vi "Mirror_GUI.vi"(10 "stop 2":refnum<vi>, 11 "GUI_cluster":T1={"Sub Panel"=refnum, "GUIdevice"="Bella_LP_Mode", "CtlRef"=refnum, "User Event in"=refnum}) -> ()   [LabVIEW 2020]
uses:
  Shared/GUI_Template/GUI_master/tcp new data cluster.ctl
  General GUIs/General-Controler/firstCall_TypDef.ctl
  Controls/eventtypdef1.ctl
  Controls/GUI_cluster.ctl
panel:
  out "UDP error message":string
  out "status ref":refnum<vi>[](array[refnum])
  out "pathRef":refnum<vi>[](array[refnum])
  in  "pushSave":bool
  out "Page Label":string="StagingTRA1"
  in  "save::4":bool caption="save"
  in  "save::3":bool caption="save"
  in  "save::2":bool caption="save"
  in  "save::1":bool caption="save"
  in  "LocalSavingPath::4":path=path "Z:/5_resources/StagingResources/TRAposition/testNEW" caption="LocalSavingPath::1"
  in  "LocalSavingPath::3":path=path "Z:/5_resources/StagingResources/TRAposition/testNEW" caption="LocalSavingPath::1"
  in  "LocalSavingPath::2":path=path "Z:/5_resources/StagingResources/TRAposition/testNEW" caption="LocalSavingPath::1"
  in  "LocalSavingPath::1":path=path "Z:/5_resources/StagingResources/TRAposition/testNEW"
  in  "save":bool
  out "GUIdevice 3":string="StagingTRA3"
  out "GUIdevice 4":string="TREX TRA1"
  out "error out":errorcluster
  out "GUIdevice 2":string="StagingTRA2"
  in  "Tab Control":T2(tab)
  in  "StepSize::1":dbl=0.01 caption="StepSize" min=-1.0 max=1.0 format="%#_2p"
  in  "Cluster 20":T3
  in  "Y":T4={"position::1"=2.74161, "Channel::1"=enum."Axis 2", "Status::1"=enum."DISABLE"} {"position::1" min=0.0 max=6.0 format="%#_8g"}
  in  "X":T5={"position::1"=3.02685, "Channel::1"=enum."Axis 1", "Status::1"=enum."DISABLE"} {"position::1" min=0.0 max=6.0 format="%#_8g"}
  in  "Cluster 40":T6
  in  "Cluster 50":T7
  in  "Cluster 30":T8
  out "device status::1":string="Initialized" caption="Device status"
  in  "<command>::1":bool
  in  "StepSize::2":dbl=0.01 caption="StepSize" min=-1.0 max=1.0 format="%#_2p"
  in  "Cluster 23":T9
  in  "Y":T10={"position::2"=3.24237, "Channel::2"=enum."Axis 2", "Status::2"=enum."DISABLE"} {"position::2" min=0.0 max=6.0 format="%#_8g"}
  in  "X":T11={"position::2"=2.27011, "Channel::2"=enum."Axis 1", "Status::2"=enum."DISABLE"} {"position::2" min=0.0 max=6.0 format="%#_8g"}
  in  "Cluster 43":T12
  in  "Cluster 53":T13
  in  "Cluster 33":T14
  out "device status::2":string="Initialized" caption="Device status"
  in  "<command>::2":bool
  in  "StepSize::3":dbl=0.01 caption="StepSize" min=-1.0 max=1.0 format="%#_2p"
  in  "Cluster 22":T15
  in  "Y":T16={"position::3"=5.00224, "Channel::3"=enum."Axis 2", "Status::3"=enum."DISABLE"} {"position::3" min=0.0 max=0.0 format="%#_8g"}
  in  "X":T17={"position::3"=1.52721, "Channel::3"=enum."Axis 1", "Status::3"=enum."DISABLE"} {"position::3" min=0.0 max=0.0 format="%#_8g"}
  in  "Cluster 42":T18
  in  "Cluster 52":T19
  in  "Cluster 32":T20
  out "device status::3":string="Initialized" caption="Device status"
  in  "<command>::3":bool
  in  "StepSize::4":dbl=0.01 caption="StepSize" min=-1.0 max=1.0 format="%#_2p"
  in  "Cluster 21":T21
  in  "Y":T22={"position::4"=4.68088, "Channel::4"=enum."Axis 2", "Status::4"=enum."DISABLE"} {"position::4" min=0.0 max=6.0 format="%#_8g"}
  in  "X":T23={"position::4"=0.99394, "Channel::4"=enum."Axis 1", "Status::4"=enum."DISABLE"} {"position::4" min=0.0 max=6.0 format="%#_8g"}
  in  "Cluster 41":T24
  in  "Cluster 51":T25
  in  "Cluster 31":T26
  out "device status::4":string="Initialized" caption="Device status"
  in  "<command>::4":bool
  in  "Mirror":T27(ring)
  out "GUIdevice 1":string="StagingTRA1"
  in  "stop":bool
  in  "Refresh Button":bool
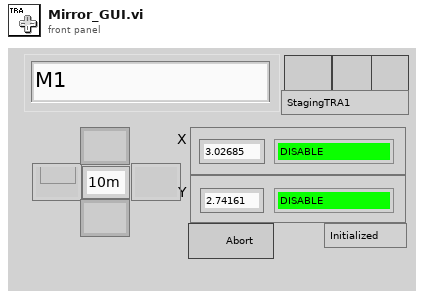
[diagram p1: front panel]
types:
  T1 = typedef "GUI_cluster.ctl" = cluster{"Sub Panel":refnum<vi>, "GUIdevice":string, "CtlRef":refnum<vi>, "User Event in":refnum<user-event>}
  T2 = enum32{"StagingTRA1", "StagingTRA2", "StagingTRA3", "TREX TRA1"}
  T3 = cluster{"relativeMovePos::1":bool, "Channel::1":enum16{"Axis 1", "Axis 3", "Axis 5"}}
  T4 = cluster{"position::1":dbl, "Channel::1":enum16{"Axis 2", "Axis 4", "Axis 6"}, "Status::1":enum16{"NOT REFERENCED", "CONFIGURATION", "HOMING", "MOVING", "READY", "DISABLE", "JOGGING"}}
  T5 = cluster{"position::1":dbl, "Channel::1":enum16{"Axis 1", "Axis 3", "Axis 5"}, "Status::1":enum16{"NOT REFERENCED", "CONFIGURATION", "HOMING", "MOVING", "READY", "DISABLE", "JOGGING"}}
  T6 = cluster{"relativeMovePos::1":bool, "Channel::1":enum16{"Axis 2", "Axis 4", "Axis 6"}}
  T7 = cluster{"relativeMoveNeg::1":bool, "Channel::1":enum16{"Axis 2", "Axis 4", "Axis 6"}}
  T8 = cluster{"relativeMoveNeg::1":bool, "Channel::1":enum16{"Axis 1", "Axis 3", "Axis 5"}}
  T9 = cluster{"relativeMovePos::2":bool, "Channel::2":enum16{"Axis 1", "Axis 3", "Axis 5"}}
  T10 = cluster{"position::2":dbl, "Channel::2":enum16{"Axis 2", "Axis 4", "Axis 6"}, "Status::2":enum16{"NOT REFERENCED", "CONFIGURATION", "HOMING", "MOVING", "READY", "DISABLE", "JOGGING"}}
  T11 = cluster{"position::2":dbl, "Channel::2":enum16{"Axis 1", "Axis 3", "Axis 5"}, "Status::2":enum16{"NOT REFERENCED", "CONFIGURATION", "HOMING", "MOVING", "READY", "DISABLE", "JOGGING"}}
  T12 = cluster{"relativeMovePos::2":bool, "Channel::2":enum16{"Axis 2", "Axis 4", "Axis 6"}}
  T13 = cluster{"relativeMoveNeg::2":bool, "Channel::2":enum16{"Axis 2", "Axis 4", "Axis 6"}}
  T14 = cluster{"relativeMoveNeg::2":bool, "Channel::2":enum16{"Axis 1", "Axis 3", "Axis 5"}}
  T15 = cluster{"relativeMovePos::3":bool, "Channel::3":enum16{"Axis 1", "Axis 3", "Axis 5"}}
  T16 = cluster{"position::3":dbl, "Channel::3":enum16{"Axis 2", "Axis 4", "Axis 6"}, "Status::3":enum16{"NOT REFERENCED", "CONFIGURATION", "HOMING", "MOVING", "READY", "DISABLE", "JOGGING"}}
  T17 = cluster{"position::3":dbl, "Channel::3":enum16{"Axis 1", "Axis 3", "Axis 5"}, "Status::3":enum16{"NOT REFERENCED", "CONFIGURATION", "HOMING", "MOVING", "READY", "DISABLE", "JOGGING"}}
  T18 = cluster{"relativeMovePos::3":bool, "Channel::3":enum16{"Axis 2", "Axis 4", "Axis 6"}}
  T19 = cluster{"relativeMoveNeg::3":bool, "Channel::3":enum16{"Axis 2", "Axis 4", "Axis 6"}}
  T20 = cluster{"relativeMoveNeg::3":bool, "Channel::3":enum16{"Axis 1", "Axis 3", "Axis 5"}}
  T21 = cluster{"relativeMovePos::4":bool, "Channel::4":enum16{"Axis 1", "Axis 3", "Axis 5"}}
  T22 = cluster{"position::4":dbl, "Channel::4":enum16{"Axis 2", "Axis 4", "Axis 6"}, "Status::4":enum16{"NOT REFERENCED", "CONFIGURATION", "HOMING", "MOVING", "READY", "DISABLE", "JOGGING"}}
  T23 = cluster{"position::4":dbl, "Channel::4":enum16{"Axis 1", "Axis 3", "Axis 5"}, "Status::4":enum16{"NOT REFERENCED", "CONFIGURATION", "HOMING", "MOVING", "READY", "DISABLE", "JOGGING"}}
  T24 = cluster{"relativeMovePos::4":bool, "Channel::4":enum16{"Axis 2", "Axis 4", "Axis 6"}}
  T25 = cluster{"relativeMoveNeg::4":bool, "Channel::4":enum16{"Axis 2", "Axis 4", "Axis 6"}}
  T26 = cluster{"relativeMoveNeg::4":bool, "Channel::4":enum16{"Axis 1", "Axis 3", "Axis 5"}}
  T27 = enum16{"M1", "BS", "M3", "OAP1", "M4", "OAP2", "M5", "n/a", "n/a ", "M20", "SIM", "M22"}
  T28 = typedef "eventtypdef1.ctl" = cluster{"label":string, "Sub Panel":refnum<vi>, "CtlRef":refnum<vi>, "This VI":refnum<vi>}
  T29 = typedef "tcp new data cluster.ctl" = cluster{"EventEnum":enum16{"new data", "connection status update"}, "Device name":string}
  T30 = typedef "firstCall_TypDef.ctl" = enum16{"reset", "read"}
  T31 = typedef "LVFontTypeDef.ctl" = cluster{"Font Name":string, "Size":u16, "Bold":bool, "Italic":bool, "Underline":bool, "Strikeout":bool, "Color":u32}
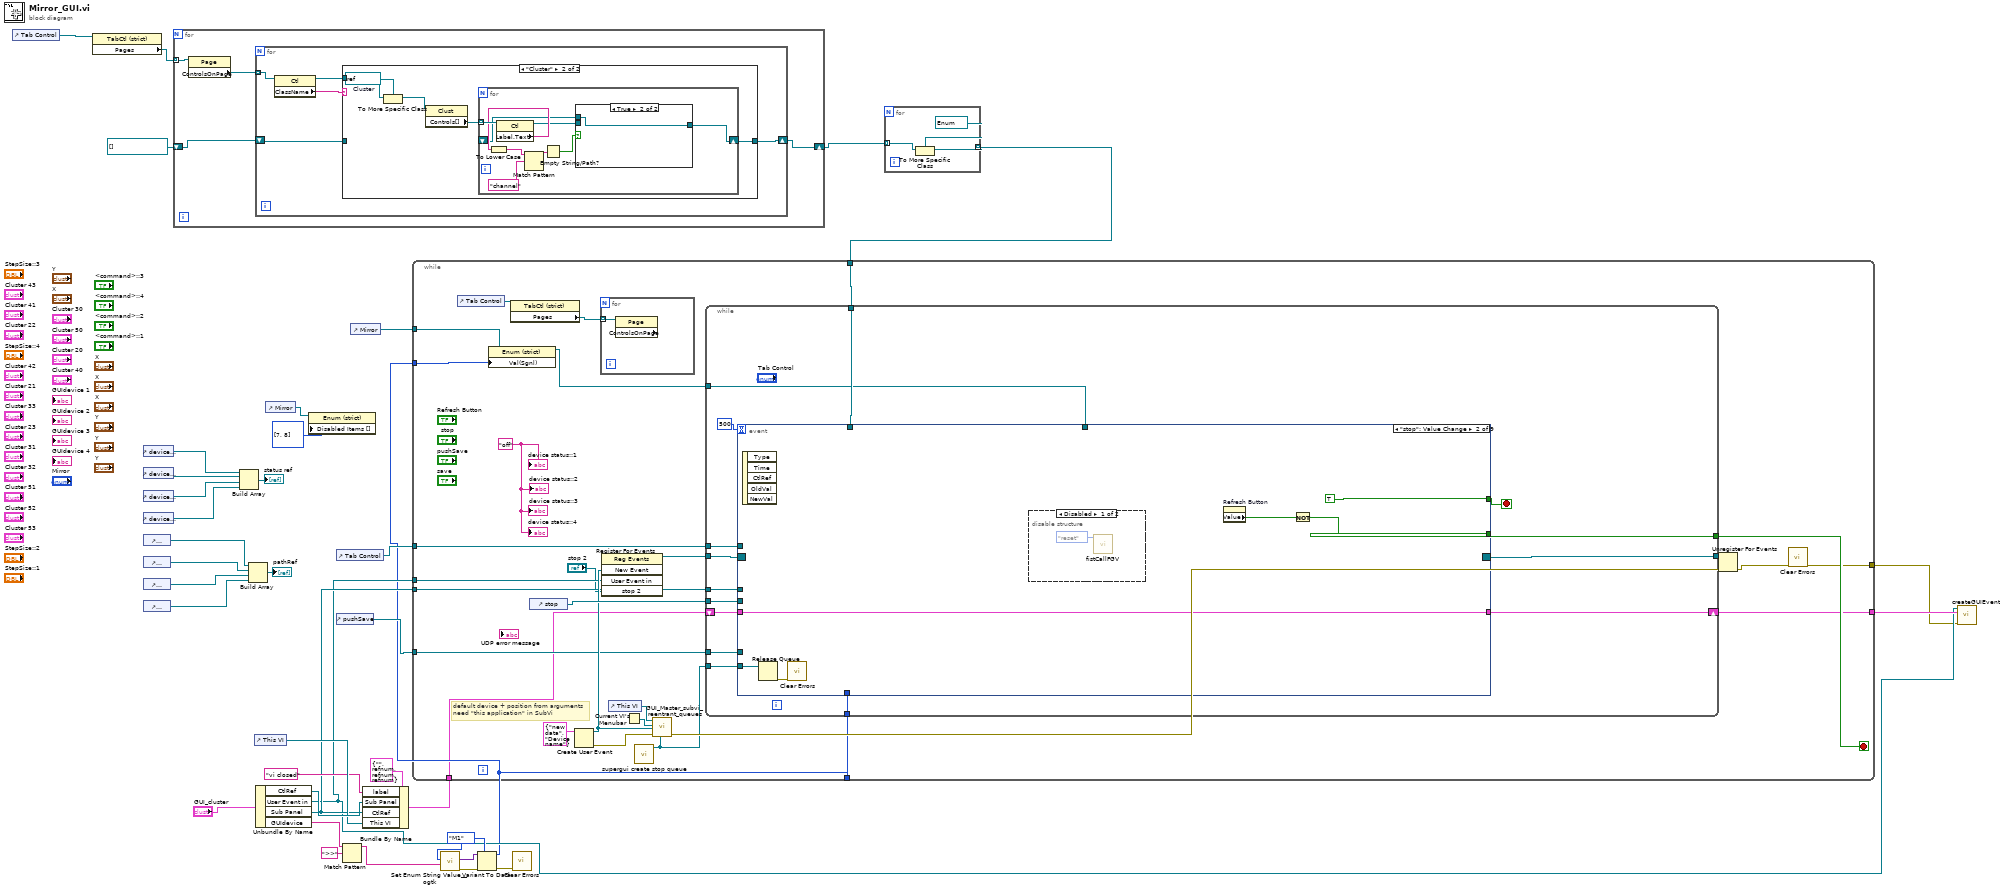
[diagram p0: block diagram]
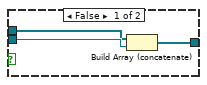
[diagram p3: hidden frame]
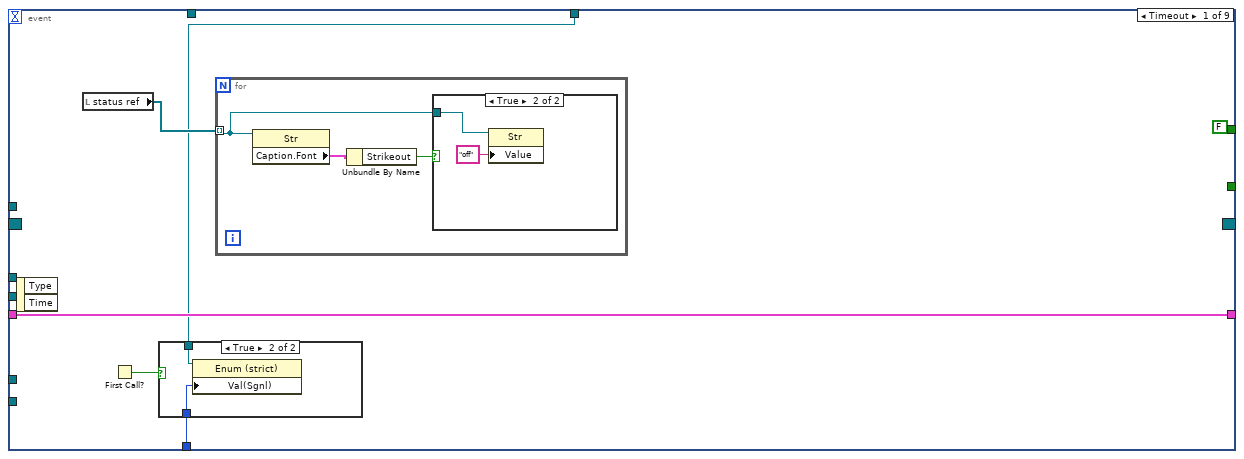
[diagram p4: hidden frame]
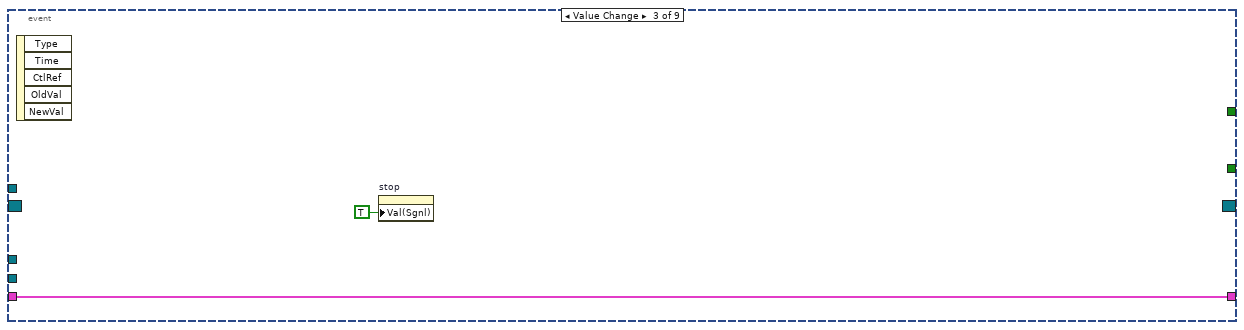
[diagram p8: hidden frame]
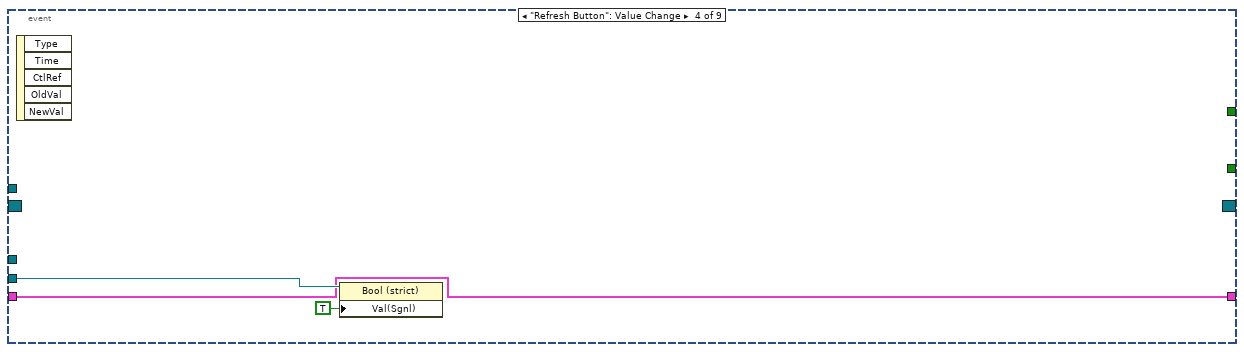
[diagram p9: hidden frame]
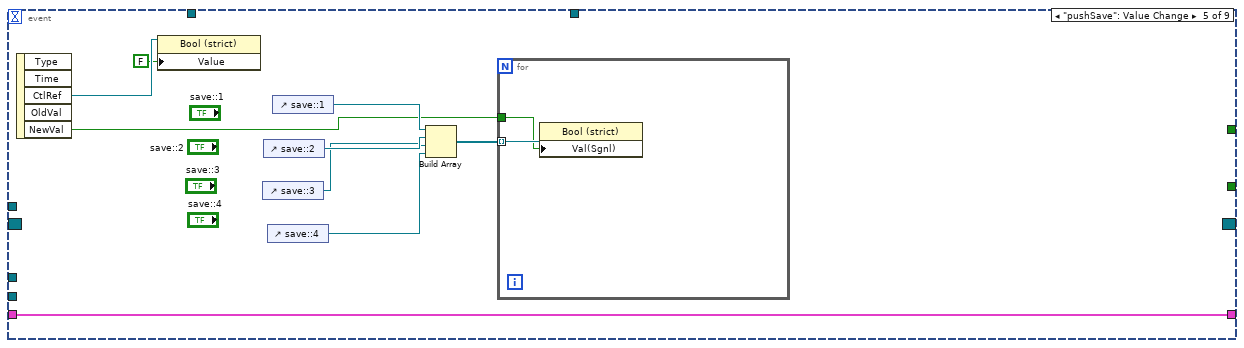
[diagram p10: hidden frame]
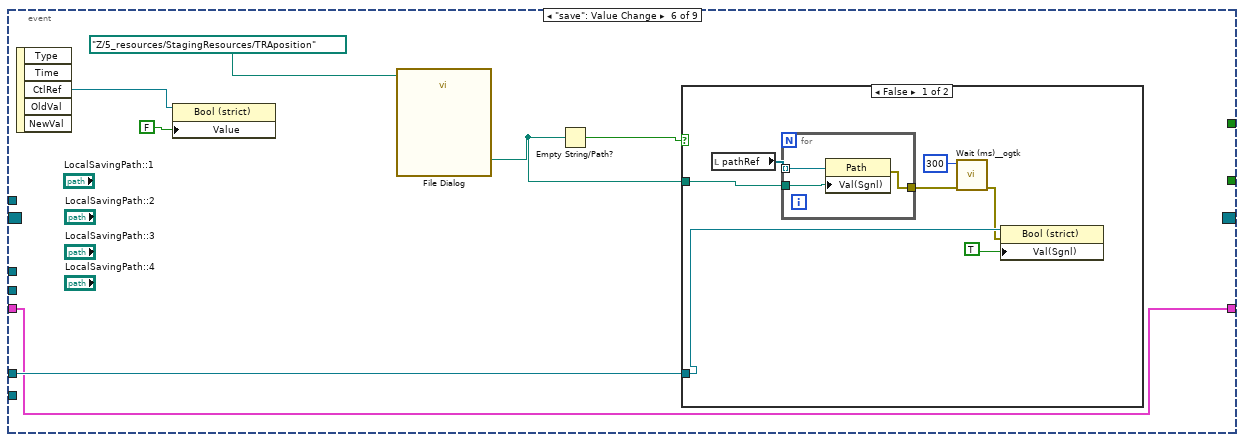
[diagram p11: hidden frame]
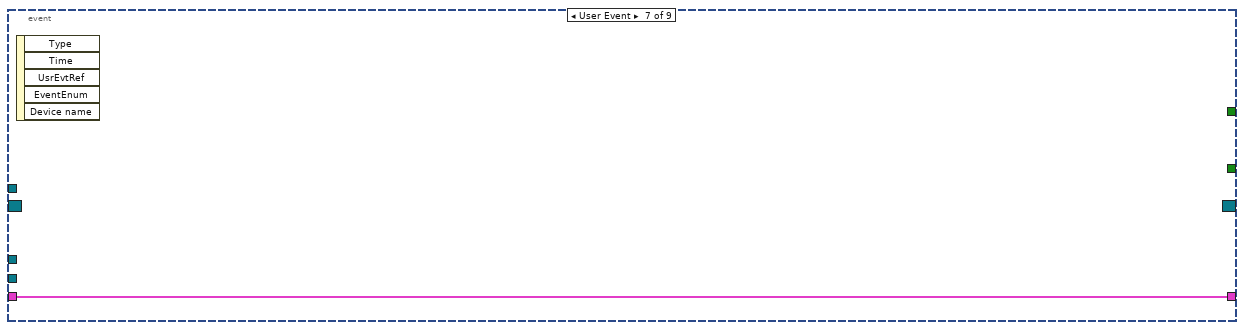
[diagram p13: hidden frame]
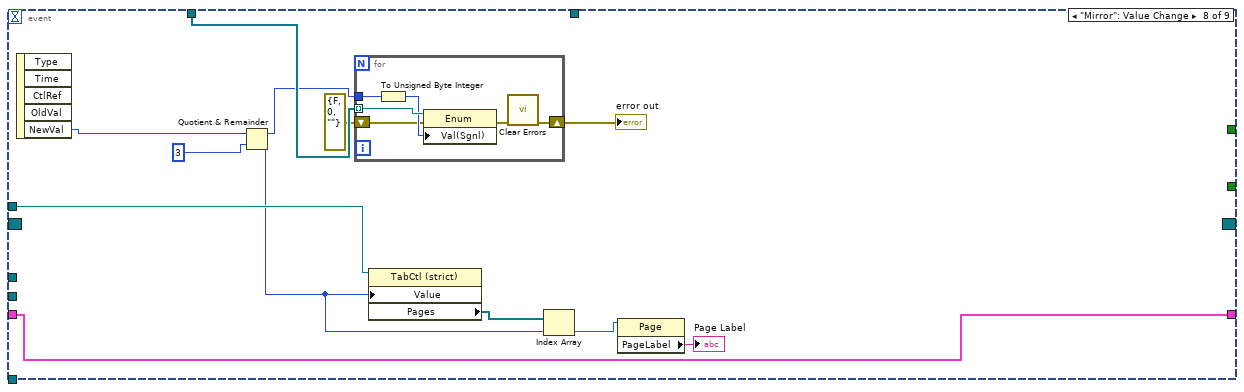
[diagram p14: hidden frame]
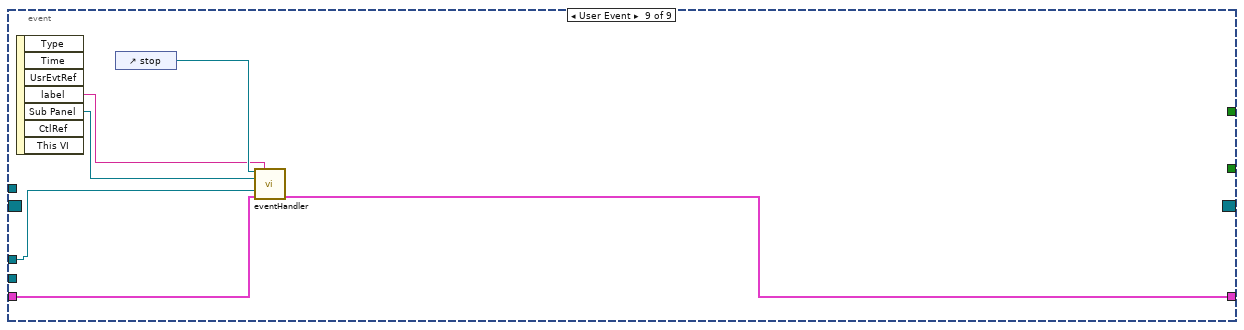
[diagram p15: hidden frame]
diagram:
  w11 = T27."M1" ("Value (Signaling)")
  n1 = control-ref of="Tab Control"() -> (w38:refnum<vi>)
  n2 = property class="TabCtl (strict)"(reference=w38) -> ("Pages"=w37:refnum<vi>[])  [unwired: 1 in, 2 out]
  n3 = control-ref of="device status::1"() -> (w23:refnum<vi>)
  n4 = control-ref of="device status::2"() -> (w22:refnum<vi>)
  n5 = control-ref of="device status::3"() -> (w21:refnum<vi>)
  n6 = control-ref of="device status::4"() -> (w20:refnum<vi>)
  n7 = control-ref of="LocalSavingPath::1"() -> (w26:refnum<vi>)
  n8 = control-ref of="LocalSavingPath::2"() -> (w27:refnum<vi>)
  n9 = control-ref of="LocalSavingPath::3"() -> (w28:refnum<vi>)
  n10 = control-ref of="LocalSavingPath::4"() -> (w29:refnum<vi>)
  n11 = for {
    tunnel: w37 -> [w42] mode=indexing
    shift-right: [w40] -> w35
    shift-left: refnum<vi>[] [] -> [w39]
    n12 = property class="Page"(reference=w42) -> ("ControlsOnPage"=w41:refnum<vi>[])  [unwired: 1 in, 2 out]
    n13 = for {
      tunnel: w41 -> [w47] mode=indexing
      shift-right: [w44] -> w40
      shift-left: w39 -> [w43]
      n14 = property class="Ctl"(reference=w47) -> (reference out=w45:refnum<vi>, "ClassName"=w46:string)  [unwired: 1 in, 1 out]
      n15 = case shown="\"Cluster\"" w46 {
        tunnel: w45 -> [_ w53]
        tunnel: [w48 w49] -> w44
        tunnel: w43 -> [w48 _]
        frame "False", Default {
        }
        frame "Cluster" {
          w52 = refnum<vi> refnum  # Cluster
          n16 = To More Specific Class(target class=w52, reference=w53) -> (specific class reference=w51:refnum<vi>)  [unwired: 1 in, 1 out]
          n17 = property class="Clust"(reference=w51) -> ("Controls[]"=w50:refnum<vi>[])  [unwired: 1 in, 2 out]
          n18 = for {
            tunnel: w50 -> [w62] mode=indexing
            shift-right: [w55] -> w49
            shift-left: _ -> [w54]
            n19 = property class="Ctl"(reference=w62) -> (reference out=w56:refnum<vi>, "Label.Text"=w60:string)  [unwired: 1 in, 1 out]
            n20 = To Lower Case(string=w60) -> (all lower case string=w59:string)
            n21 = Match Pattern(string=w59, regular expression="channel") -> (match substring=w58:string)  [unwired: 1 in, 3 out]
            n22 = Empty String/Path?(string/path=w58) -> (empty?=w57:bool)
            n23 = case shown="True" w57 {
              tunnel: w56 -> [w65 _]
              tunnel: [w64 w66] -> w55
              tunnel: w54 -> [w63 w66]
              frame False {
                n24 = Build Array (concatenate)(w63, w65) -> (w64:refnum<vi>[])
              }
              frame True {
              }
            }
          }
        }
      }
    }
  }
  n25 = Build Array(w23, w22, w21, w20) -> (→"status ref":refnum<vi>[])
  n26 = Build Array(w26, w27, w28, w29) -> (→"pathRef":refnum<vi>[])
  n27 = control-ref of="This VI"() -> (w16:refnum<vi>)
  n28 = Unbundle By Name("GUI_cluster") -> ("CtlRef"=w17:refnum<vi>, "User Event in"=w3:refnum<user-event>, "Sub Panel"=w6:refnum<vi>, "GUIdevice"=w14:string)
  n29 = control-ref of="Mirror"() -> (w31:refnum<vi>)
  n30 = property class="Enum (strict)"(reference=w31, "Disabled Items []"=i32[] [7, 8]) -> ()  [unwired: 1 in, 2 out]
  n31 = control-ref of="Tab Control"() -> (w33:refnum<vi>)
  n32 = control-ref of="pushSave"() -> (w24:refnum<vi>)
  n33 = Match Pattern(string=w14, regular expression=">>") -> (before substring=w8:string)  [unwired: 1 in, 3 out]
  n34 = control-ref of="Mirror"() -> (w30:refnum<vi>)
  n35 = Bundle By Name(cluster=T28 {"label"="", "Sub Panel"=refnum, "CtlRef"=refnum, "This VI"=refnum} ("event data"), "label"="vi closed", "Sub Panel"=w6, "CtlRef"=w17, "This VI"=w16) -> (w4:T28)
  n36 = call <userlib>:"Set Enum String Value__ogtk.vi"("String Value"=w8, "Default Enum Value"=w11) -> ("error out"=w9:errorcluster, "Enum"=w12:variant)  [unwired: 8 in]
  n37 = Variant To Data(error in=w9, type=w11, Variant=w12) -> (data=w1:T27, error out=w10:errorcluster)
  n38 = call <vilib>:"Clear Errors.vi"("error in (no error)"=w10) -> ()  [unwired: 5 in, 2 out]
  n39 = for {
    tunnel: w35 -> [w69] mode=indexing
    tunnel: [w68] -> w34 mode=indexing
    n40 = To More Specific Class(target class=refnum<vi> refnum ("Channel::2"), reference=w69) -> (specific class reference=w68:refnum<vi>)  [unwired: 1 in, 1 out]
  }
  n41 = while {
    tunnel: w34 -> [w84]
    tunnel: w33 -> [w83]
    tunnel: w30 -> [w82]
    tunnel: w24 -> [w81]
    tunnel: [w79] -> w2
    tunnel: w3 -> [w78]
    tunnel: w1 -> [w77]
    tunnel: w6 -> [w76]
    tunnel: w4 -> [w74]
    tunnel: [w73] -> w5
    tunnel: w1 -> [w71]
    stop <- w95 stop-if-true
    w80 = "off" ("device status::1")
    # "default device + position from arguments\nneed \"this application\" in SubVi"
    n42 = control-ref of="Tab Control"() -> (w86:refnum<vi>)
    n43 = property class="Enum (strict)"(reference=w82, "Val(Sgnl)"=w77) -> (reference out=w75:refnum<vi>)  [unwired: 1 in, 1 out]
    n44 = property class="TabCtl (strict)"(reference=w86) -> ("Pages"=w85:refnum<vi>[])  [unwired: 1 in, 2 out]
    n45 = control-ref of="stop"() -> (w94:refnum<vi>)
    n46 = Create User Event(user event datatype=T29 {"EventEnum"=enum."new data", "Device name"="Device name"} ("New Event")) -> (user event=w89:refnum<user-event>, error out=w90:errorcluster)  [unwired: 1 in]
    n47 = for {
      tunnel: w85 -> [w98] mode=indexing
      n48 = property class="Page" props=["ControlsOnPage"](reference=w98) -> ()  [unwired: 1 in, 3 out]
    }
    n49 = register-events(w89, w78, "stop 2") -> (reference out=w97:refnum<event-registration>)  [unwired: 2 in, 1 out]
    n50 = control-ref of="This VI"() -> (w93:refnum<vi>)
    n51 = Current VI's Menubar() -> (w92:refnum<k9>)
    n52 = call "supergui create stop queue.vi"() -> ("STOP Queue out"=w70:refnum<queue>)  [unwired: 11 in]
    n53 = call "GUI_Master_subvi_reentrant_queues.vi"("STOP Queue in"=w70, "error in (no error)"=w90, "tcp data event"=w89, "Caller menu reference"=w92, "Caller VI ref"=w93) -> ("error out"=w88:errorcluster)  [unwired: 6 in]
    n54 = while {
      tunnel: w97 -> [w113]
      tunnel: [w112] -> w96
      tunnel: [w110] -> w95
      tunnel: w94 -> [w109]
      tunnel: w84 -> [w108]
      tunnel: w83 -> [w107]
      tunnel: w81 -> [w106]
      tunnel: w76 -> [w104]
      tunnel: w75 -> [w103]
      shift-right: [w101] -> w73
      shift-left: w74 -> [w102]
      tunnel: w71 -> [w100]
      tunnel: w70 -> [w99]
      stop <- w111 stop-if-true
      n55 = event shown="[1] \"stop\": Value Change" {
        selector: w113 -> [_ _ _ _ _ _ _ _ _]
        dyn-events: [_ _ _ _ _ _ _ _ _] -> w112
        timeout: 500 -> [_ _ _ _ _ _ _ _ _]
        tunnel: [FALSE TRUE _ _ _ _ _ _ _] -> w111
        tunnel: [_ w130 _ _ _ _ _ _ _] -> w110
        tunnel: w109 -> [_ _ _ w138 _ _ _ _ _]
        tunnel: w108 -> [_ _ _ _ _ _ _ w179 _]
        tunnel: w107 -> [_ _ _ _ _ _ _ w173 _]
        tunnel: w106 -> [_ _ _ _ _ w153 _ _ _]
        tunnel: w104 -> [_ _ _ _ _ _ _ _ w188]
        tunnel: w103 -> [w116 _ _ _ _ _ _ _ _]
        tunnel: w102 -> [w117 w129 w135 w136 w139 w150 w167 w168 w187]
        tunnel: [w117 w129 w135 w136 w139 w150 w167 w168 w186] -> w101
        tunnel: w100 -> [w115 _ _ _ _ _ _ _ _]
        tunnel: w99 -> [_ w128 _ _ _ _ _ _ _]
        event Timeout {
          n56 = event-data() -> ()  [unwired: 1 in, 2 out]
          n57 = local read "status ref"() -> (w118:refnum<vi>[])
          n58 = First Call?() -> (First Call?: T/F=w114:bool)
          n59 = case shown="True" w114 {
            tunnel: w116 -> [_ w121]
            tunnel: w115 -> [_ w120]
            frame False {
            }
            frame True {
              n60 = property class="Enum (strict)"(reference=w121, "Val(Sgnl)"=w120) -> ()  [unwired: 1 in, 2 out]
            }
          }
          n61 = for {
            tunnel: w118 -> [w122] mode=indexing
            n62 = property class="Str"(reference=w122) -> ("Caption.Font"=w124:T31)  [unwired: 1 in, 2 out]
            n63 = Unbundle By Name(w124) -> ("Strikeout"=w123:bool)
            n64 = case shown="True" w123 {
              tunnel: w122 -> [_ w126]
              frame False {
              }
              frame True {
                n65 = property class="Str"(reference=w126, "Value"="off") -> ()  [unwired: 1 in, 2 out]
              }
            }
          }
        }
        event "stop": Value Change {
          n66 = event-data() -> ()  [unwired: 1 in, 5 out]
          n67 = Release Queue(queue=w128) -> (error out=w127:errorcluster)  [unwired: 2 in, 2 out]
          n68 = call <vilib>:"Clear Errors.vi"("error in (no error)"=w127) -> ()  [unwired: 5 in, 2 out]
          n69 = disable-structure shown="Disabled" {
            frame Disabled {
              n70 = call "fistCallFGV.vi"("Function"=firstCall_TypDef."reset") -> ()  [unwired: 9 in, 2 out]
            }
            frame Enabled {
            }
          }
          n71 = property on="Refresh Button" class="Bool (strict)"() -> ("Value"=w131:bool)  [unwired: 2 in, 2 out]
          n72 = Not(x=w131) -> (.not. x?=w130:bool)
        }
        event Value Change {
          n73 = event-data() -> ()  [unwired: 1 in, 5 out]
          n74 = property on="stop" class="Bool (strict)"("Val(Sgnl)"=TRUE ("Value (Signaling)")) -> ()  [unwired: 2 in, 2 out]
        }
        event "Refresh Button": Value Change {
          n75 = event-data() -> ()  [unwired: 1 in, 5 out]
          n76 = property class="Bool (strict)"(reference=w138, "Val(Sgnl)"=TRUE ("Value (Signaling)")) -> ()  [unwired: 1 in, 2 out]
        }
        event "pushSave": Value Change {
          n77 = event-data() -> ("CtlRef"=w141:refnum<vi>, "NewVal"=w142:bool)  [unwired: 1 in, 3 out]
          n78 = property class="Bool (strict)"(reference=w141, "Value"=FALSE) -> ()  [unwired: 1 in, 2 out]
          n79 = control-ref of="save::3"() -> (w145:refnum<vi>)
          n80 = control-ref of="save::2"() -> (w146:refnum<vi>)
          n81 = control-ref of="save::4"() -> (w144:refnum<vi>)
          n82 = control-ref of="save::1"() -> (w147:refnum<vi>)
          n83 = Build Array(w147, w146, w145, w144) -> (w143:refnum<vi>[])
          n84 = for {
            tunnel: w143 -> [w149] mode=indexing
            tunnel: w142 -> [w148]
            n85 = property class="Bool (strict)"(reference=w149, "Val(Sgnl)"=w148) -> ()  [unwired: 1 in, 2 out]
          }
        }
        event "save": Value Change {
          n86 = event-data() -> ("CtlRef"=w152:refnum<vi>)  [unwired: 1 in, 4 out]
          n87 = property class="Bool (strict)"(reference=w152, "Value"=FALSE) -> ()  [unwired: 1 in, 2 out]
          n88 = call "File Dialog"("start path"=path "Z:/5_resources/StagingResources/TRAposition") -> ("selected path"=w155:path)  [unwired: 11 in, 3 out]
          n89 = Empty String/Path?(string/path=w155) -> (empty?=w154:bool)
          n90 = case shown="False" w154 {
            tunnel: w155 -> [w163 _]
            tunnel: w153 -> [w159 _]
            frame False {
              n91 = local read "pathRef"() -> (w162:refnum<vi>[])
              n92 = for {
                tunnel: w162 -> [w166] mode=indexing
                tunnel: w163 -> [w165]
                tunnel: [w164] -> w161
                n93 = property class="Path"(reference=w166, "Val(Sgnl)"=w165) -> (error out=w164:errorcluster)  [unwired: 1 in, 1 out]
              }
              n94 = call <userlib>:"Wait (ms)__ogtk.vi"("error in (no error)"=w161, "milliseconds to wait"=u32 300) -> ("error out"=w158:errorcluster)  [unwired: 8 in, 1 out]
              n95 = property class="Bool (strict)"(reference=w159, error in=w158, "Val(Sgnl)"=TRUE) -> ()  [unwired: 2 out]
            }
            frame True {
            }
          }
        }
        event User Event {
          n96 = event-data() -> ()  [unwired: 1 in, 5 out]
        }
        event "Mirror": Value Change {
          n97 = event-data() -> ("NewVal"=w178:T27)  [unwired: 1 in, 4 out]
          n98 = Quotient & Remainder(x=w178, y=3) -> (x-y*floor(x/y)=w176:i32, floor(x/y)=w171:i32)
          n99 = for {
            tunnel: w179 -> [w185] mode=indexing
            tunnel: w176 -> [w183]
            shift-right: [w181] -> w174
            shift-left: errorcluster {"status"=FALSE, "code"=0, "source"=""} ("error out") -> [w180]
            n100 = To Unsigned Byte Integer(number=w183) -> (unsigned 8bit integer=w182:u8)
            n101 = property class="Enum"(reference=w185, error in=w180, "Val(Sgnl)"=w182) -> (error out=w184:errorcluster)  [unwired: 1 out]
            n102 = call <vilib>:"Clear Errors.vi"("error in (no error)"=w184) -> ("error out"=w181:errorcluster)  [unwired: 5 in, 1 out]
          }
          "error out" <- w174
          n103 = property class="TabCtl (strict)"(reference=w173, "Value"=w171) -> ("Pages"=w172:refnum<vi>[])  [unwired: 1 in, 2 out]
          n104 = Index Array(array=w172, index=w171) -> (element=w170:refnum<vi>)
          n105 = property class="Page"(reference=w170) -> ("PageLabel"=→"Page Label":string)  [unwired: 1 in, 2 out]
        }
        event User Event {
          n106 = event-data() -> ("label"=w190:string, "Sub Panel"=w189:refnum<vi>)  [unwired: 1 in, 5 out]
          n107 = control-ref of="stop"() -> (w191:refnum<vi>)
          n108 = call "eventHandler.vi"("Boolean in"=w191, "label"=w190, "Sub Panel 2"=w189, "Sub Panel"=w188, "event data in"=w187) -> ("event data out"=w186:T28)  [unwired: 10 in]
        }
      }
    }
    n109 = Unregister For Events(event registration refnum=w96, error in=w88) -> (error out=w87:errorcluster)
    n110 = call <vilib>:"Clear Errors.vi"("error in (no error)"=w87) -> ("error out"=w79:errorcluster)  [unwired: 5 in, 1 out]
    "device status::1" <- w80
    "device status::2" <- w80
    "device status::3" <- w80
    "device status::4" <- w80
  }
  n111 = call "createGUIEvent.vi"("error in (no error)"=w2, "event data"=w5, "User Event in"=w3) -> ()  [unwired: 8 in, 1 out]
